vi "StopSignal-TestMain5.vi"() -> ()   [LabVIEW 2017]
uses:
  StopSignal.lvlib
panel:
  out "error out":errorcluster
  out "reason #4":string
  out "timestamp #4":timestamp
  out "reason #3":string
  out "timestamp #3":timestamp
  out "reason #2":string
  out "timestamp #2":timestamp
  in  "stop":bool
  out "reason #1":string
  out "timestamp #1":timestamp
  out "current time":timestamp
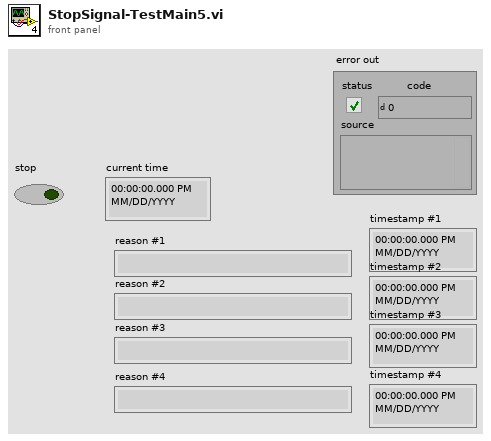
[diagram p1: front panel]
types:
  T1 = typedef "StopSignal.lvlib/StopSignal.ctl" = refnum<k1>
  T2 = typedef "StopSignal.lvlib/def-StopReason.ctl" = cluster{"Reason":string, "timestamp":timestamp}
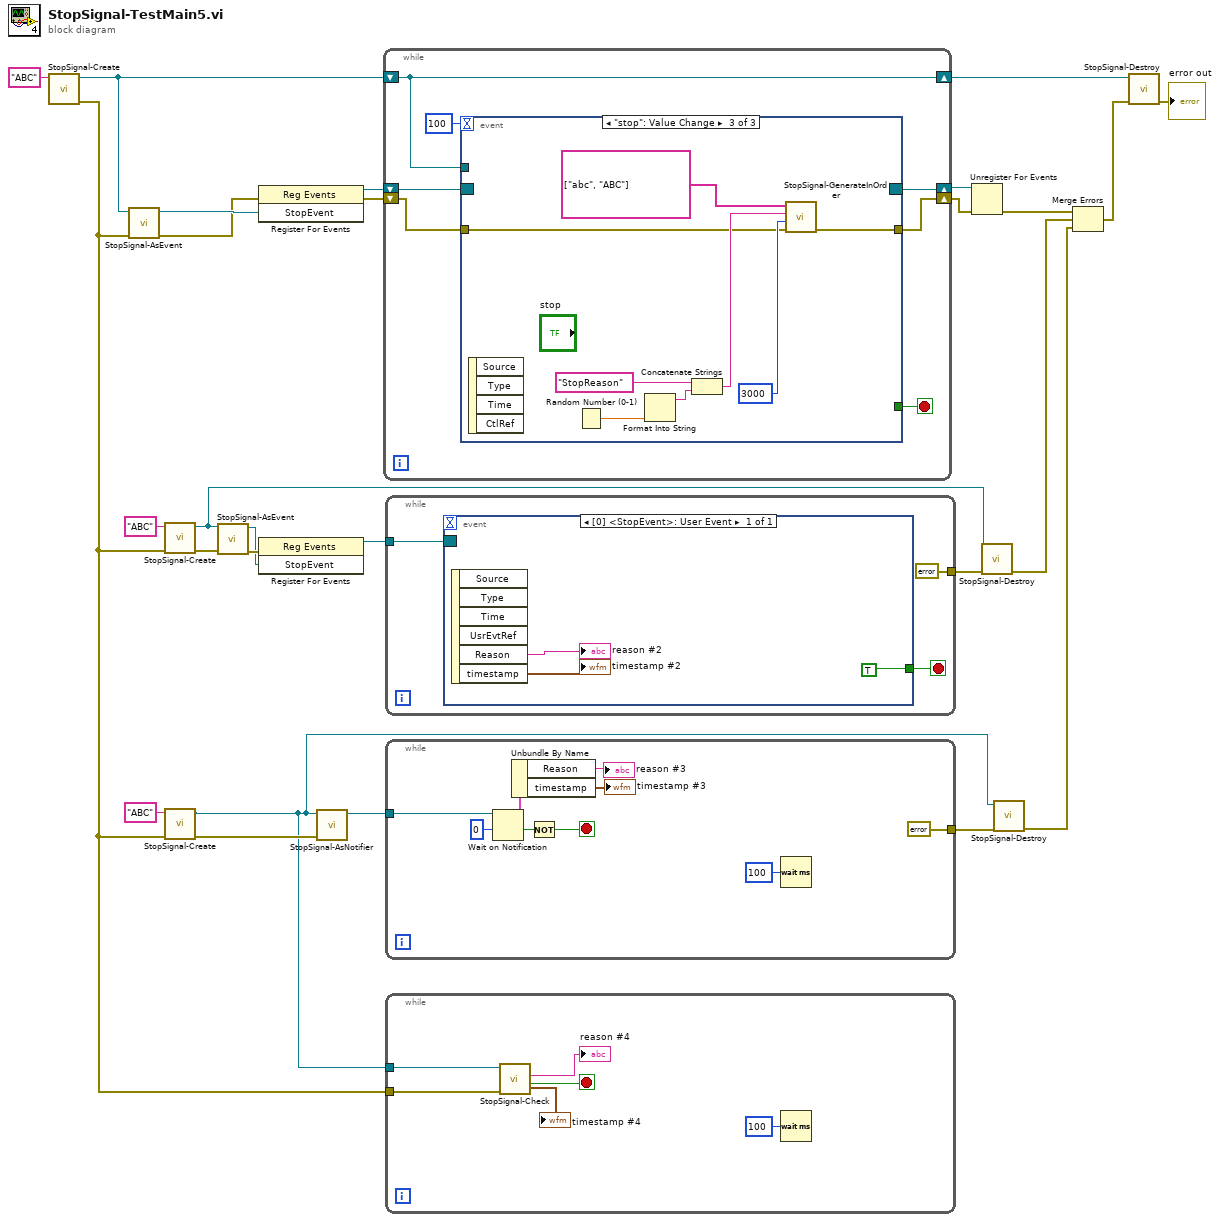
[diagram p0: block diagram]
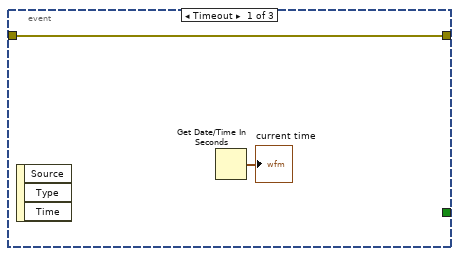
[diagram p2: hidden frame]
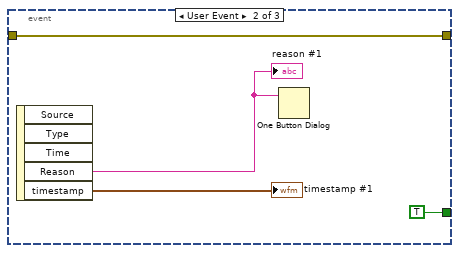
[diagram p3: hidden frame]
diagram:
  n1 = call "StopSignal-Create.vi"("name(\"\")"="ABC" ("name(\"\")")) -> ("error out"=w11:errorcluster, "StopSignal"=w20:T1)  [unwired: 9 in]
  n2 = call "StopSignal-AsEvent.vi"("error in (no error)"=w11, "StopSignal"=w20) -> ("error out"=w4:errorcluster, "StopEvent"=w23:refnum<user-event>)  [unwired: 8 in]
  n3 = call "StopSignal-Create.vi"("error in (no error)"=w11, "name(\"\")"="ABC" ("name(\"\")")) -> ("error out"=w17:errorcluster, "StopSignal"=w14:T1)  [unwired: 8 in]
  n4 = call "StopSignal-Create.vi"("error in (no error)"=w11, "name(\"\")"="ABC" ("name(\"\")")) -> ("error out"=w10:errorcluster, "StopSignal"=w9:T1)  [unwired: 8 in]
  n5 = call "StopSignal-AsEvent.vi"("error in (no error)"=w17, "StopSignal"=w14) -> ("error out"=w16:errorcluster, "StopEvent"=w15:refnum<user-event>)  [unwired: 8 in]
  n6 = register-events(error in=w4, w23) -> (reference out=w27:refnum<event-registration>, error out=w3:errorcluster)  [unwired: 1 in]
  n7 = register-events(error in=w16, w15) -> (reference out=w25:refnum<event-registration>)  [unwired: 1 in, 1 out]
  n8 = call "StopSignal-AsNotifier.vi"("error in (no error)"=w10, "StopSignal"=w9) -> ("StopNotifier"=w21:refnum<notifier>)  [unwired: 8 in, 1 out]
  n9 = while {
    shift-right: [w31] -> w26
    shift-left: w27 -> [w34]
    shift-right: [w30] -> w22
    shift-left: w20 -> [w30]
    shift-right: [w28] -> w2
    shift-left: w3 -> [w29]
    stop <- w33 stop-if-true
    n10 = event shown="[2] \"stop\": Value Change" {
      selector: w34 -> [_ _ _]
      dyn-events: [_ _ _] -> w31
      timeout: 100 -> [_ _ _]
      tunnel: [_ TRUE _] -> w33
      tunnel: w30 -> [_ _ _]
      tunnel: w29 -> [w35 w37 w42]
      tunnel: [w35 w37 w41] -> w28
      event Timeout {
        n11 = event-data() -> ()  [unwired: 1 in, 3 out]
        n12 = Get Date/Time In Seconds() -> (seconds since 1Jan1904=→"current time":timestamp)
      }
      event User Event {
        n13 = event-data() -> ("Reason"=w39:string, "timestamp"=→"timestamp #1":timestamp)  [unwired: 1 in, 3 out]
        "reason #1" <- w39
        n14 = One Button Dialog(message=w39) -> ()  [unwired: 1 in, 1 out]
      }
      event "stop": Value Change {
        n15 = event-data() -> ()  [unwired: 1 in, 4 out]
        n16 = Random Number (0-1)() -> (number: 0 to 1=w47:dbl)
        n17 = Format Into String(w47) -> (resulting string=w46:string)  [unwired: 3 in, 1 out]
        n18 = Concatenate Strings("StopReason" ("event data"), w46) -> (w45:string)
        n19 = call "StopSignal-GenerateInOrder.vi"("error in (no error)"=w42, "interval time(ms)"=u32 3000, "reason(\"\")"=w45, "name(\"\")"=string[] ["abc", "ABC"] ("name(\"\")")) -> ("error out"=w41:errorcluster)  [unwired: 7 in]
      }
    }
  }
  n20 = while {
    tunnel: w25 -> [w51]
    tunnel: [errorcluster {"status"=FALSE, "code"=0, "source"=""} ("error out")] -> w13
    stop <- w50 stop-if-true
    n21 = event shown="[0] <StopEvent>: User Event" {
      selector: w51 -> [_]
      dyn-events: _ -> [_]
      timeout: _ -> [_]
      tunnel: [TRUE] -> w50
      event User Event {
        n22 = event-data() -> ("Reason"=→"reason #2":string, "timestamp"=→"timestamp #2":timestamp)  [unwired: 1 in, 4 out]
      }
    }
  }
  n23 = while {
    tunnel: w21 -> [w59]
    tunnel: [errorcluster {"status"=FALSE, "code"=0, "source"=""} ("error out")] -> w8
    stop <- w60 stop-if-true
    n24 = Wait on Notification(notifier=w59, timeout in ms (-1)=0) -> (notification=w58:T2, timed out?=w62:bool)  [unwired: 2 in, 2 out]
    n25 = Unbundle By Name(w58) -> ("Reason"=→"reason #3":string, "timestamp"=→"timestamp #3":timestamp)
    n26 = Not(x=w62) -> (.not. x?=w60:bool)
    n27 = Wait (ms)(milliseconds to wait=u32 100) -> ()  [unwired: 1 out]
  }
  n28 = while {
    tunnel: w9 -> [w68]
    tunnel: w11 -> [w67]
    stop <- w66 stop-if-true
    n29 = call "StopSignal-Check.vi"("error in (no error)"=w67, "StopSignal"=w68) -> ("Stop?"=w66:bool, "Reason"=→"reason #4":string, "timestamp"=→"timestamp #4":timestamp)  [unwired: 5 in, 2 out]
    n30 = Wait (ms)(milliseconds to wait=u32 100) -> ()  [unwired: 1 out]
  }
  n31 = Unregister For Events(event registration refnum=w26, error in=w2) -> (error out=w24:errorcluster)
  n32 = call "StopSignal-Destroy.vi"("error in (no error)"=w13, "StopSignal"=w14) -> ("error out"=w6:errorcluster)  [unwired: 9 in]
  n33 = call "StopSignal-Destroy.vi"("error in (no error)"=w8, "StopSignal"=w9) -> ("error out"=w5:errorcluster)  [unwired: 9 in]
  n34 = Merge Errors(w24, w6, w5) -> (w7:errorcluster)
  n35 = call "StopSignal-Destroy.vi"("error in (no error)"=w7, "StopSignal"=w22) -> ("error out"=→"error out":errorcluster)  [unwired: 9 in]
